vi "StartProgram.vi"(8 "error in (no error)":errorcluster, 11 "FPGA VI Reference In":refnum<k20>) -> (0 "error out":errorcluster, 3 "FPGA VI Reference out":refnum<k20>)   [LabVIEW 2018]
uses:
  Type_Def/Type_Def ControlState.ctl
  Type_Def/Type_Def Master_DataControls.ctl
  Type_Def/TypeDef_cRIODatas.ctl
  Type_Def/Type_Def IMUDatas.ctl
  Type_Def/TypeDef_BMSDatas.ctl
  Type_Def/TypeDef_BMSStatuss.ctl
  Type_Def/TypeDef FixedMotorData.ctl
  Type_Def/Type_Def Actuator Controls.ctl
  Type_Def/TypeDef_MotorData.ctl
  Type_Def/TypeDef_LoopPeriod.ctl
  Type_Def/Master_DataControl.ctl
  <vilib>/Utility/error.llb/Error Cluster From Error Code.vi
  <vilib>/rvi/errors/niLvFpgaAdjustHostInterfaceError.vi
  <vilib>/rvi/interface/nirviReadWriteControl/nirviReadWriteControl.xnode
  <vilib>/NI_Real-Time Target Support.lvlib
  NiFpgaLv.dll
  <vilib>/rvi/interface/Simulation/niFpgaSimulationCallBeginRW.vi
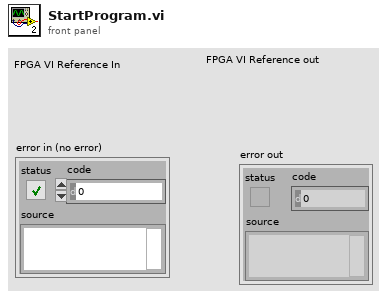
[diagram p1: front panel]
types:
  T1 = cluster{"x acceleration (g)":dbl, "Pressure (psia)":dbl, "Temperature (F)":dbl}
  T2 = typedef "Type_Def Master_DataControls.ctl" = cluster{"cRIO Data":T3, "IMU Data":T4, "BMS Data":T5, "Motor Data":T7}
  T3 = typedef "TypeDef_cRIODatas.ctl" = cluster{"HallEffect Right (cm)":dbl, "HallEffect Left (cm)":dbl, "Optical Sensor 1 (V)":dbl, "Optical Sensor 2 (V)":dbl, "24V Voltage  (V)":dbl, "24V Current (A)":dbl, "Contactor H1 Continuity":dbl, "Contactor L1 Continuity ":dbl, "Contactor H2 Continuity":dbl, "Contactor L2 Continuity ":dbl, "Brake PT(psig)":dbl, "Pump PT (psig)":dbl, "24V Temp   (C)":dbl, "Tank PT(psig) ":dbl, "ABS Pressure 1 (psig)":dbl, "ABS Pressure 2 (psig) ":dbl, "Displacement (ft)":dbl, "Velocity (ft/s)":dbl, "Time (ms)":dbl, "PV 1 Temp":dbl, "PV2 Temp":dbl}
  T4 = typedef "Type_Def IMUDatas.ctl" = cluster{"x acceleration (g)":dbl, "Pressure (psia)":dbl, "Temperature (F)":dbl}
  T5 = typedef "TypeDef_BMSDatas.ctl" = cluster{"Pack 1 Max Cell\n Voltage (V)":dbl, "Pack 1 Max Cell\n ID ":dbl, "Pack 1 Min Cell \nVoltage (V)":dbl, "Pack 1 Min Cell \nID ":dbl, "Pack 1 State of Charge  (%)":dbl, "Pack 1 Average Voltage1 (V)":dbl, "Pack 1Voltage Delta (V)":dbl, "Pack 1 Current (A)":dbl, "Pack 1 Voltage (V)":dbl, "Pack 1 Max Resistance (Ohm)":dbl, "Pack 1Min Resistance (Ohm)":dbl, "Pack 1Average Resistance (Ohm)":dbl, "Pack 1Delta Resistance (Ohm)":dbl, "Pack 1 Highest Temperature(F)":dbl, "BmsStatus1":T6, "Pack 2 Max Cell\n Voltage (V) ":dbl, "Pack 2 Max Cell\n ID  ":dbl, "Pack 2 Min Cell \nVoltage (V) ":dbl, "Pack 2 Min Cell \nID  ":dbl, "Pack 2 Average Voltage1 (V)":dbl, "Pack 2 Voltage Delta (V) ":dbl, "Pack 2 Current (A)":dbl, "Pack 2 Voltage (V) ":dbl, "Pack 2 State of Charge  (%) ":dbl, "Pack 2 Max Resistance (Ohm) ":dbl, "Pack 2 Min Resistance (Ohm)":dbl, "Pack 2 Average Resistance (Ohm)":dbl, "Pack 2 Delta Resistance (Ohm) ":dbl, "Pack 2 Highest Temperature(F) ":dbl, "BmsStatus 2":T6}
  T6 = typedef "TypeDef_BMSStatuss.ctl" = cluster{"isFault":bool, "isolationMonitoring":bool}
  T7 = typedef "TypeDef FixedMotorData.ctl" = cluster{" Velocity (RPM)":dbl, " MotorTemp(C)":dbl, " ControlTemp(C)":dbl, " DcLinkVolt(V)":dbl, " ErrorCode":dbl, "IsAlive":bool, "motorStatus":cluster{"isReady":bool, "isOn":bool, "isOperEn":bool, "isFault":bool, "isVoltEn":bool, "targetReached":bool, "isWarning":bool}, "motorControllerState":u16}
  T8 = typedef "TypeDef_MotorData.ctl" = cluster{" Velocity (RPM)":i32, " MotorTemp(C)":u8, " ControlTemp(C)":u8, " DcLinkVolt(V)":dbl, " ErrorCode":dbl, "IsAlive":bool, "motorStatus":cluster{"isReady":bool, "isOn":bool, "isOperEn":bool, "isFault":bool, "isVoltEn":bool, "targetReached":bool, "isWarning":bool}, "motorControllerState":u16}
  T9 = typedef "Type_Def Actuator Controls.ctl" = cluster{"Reverse ":bool, "Precharge Ctrl":bool, "Pump Ctrl":bool, "24 VDC Ctr":bool, "Vent Solenoid":bool, "Brake Solenoid":bool, "EMCY  Brake Solenoid":bool, "Digital Out 7B ":bool, "Forward Ctrl":bool, "Contact H1":bool, "Contact L1":bool, "Contact H2":bool, "Contact L2 ":bool, "LED RED":bool, "LED GREEN":bool, " Digital Out 7A":bool}
  T10 = typedef "Type_Def ControlState.ctl" = enum16{"Blank", "Systems Check", "Idle", "Ready", "Pushing", "CrawlingPrecharge", "Braking", "Fault", "Boot Up", "Unpowered", "Crawling", "Shutdown", "Service Push", "Service Wait", "Vent", "Precharge"}
  T11 = cluster{"Forward":bool, "Low Side":bool, "Precharge":bool, "High Side":bool, "Digital Out 5":bool, "Digital Out 6":bool, "Digital Out 7 ":bool, "24 Power":bool, "Tank Valve ":bool, "Brake Valve":bool, "Pump":bool, "Digital Out 1 ":bool, "Digital Out 2":bool, "Digital Out 3":bool, "Digital Out 4 ":bool, "Reverse":bool}
  T12 = typedef "TypeDef_LoopPeriod.ctl" = cluster{"Control Period":i64, "DAQ Period":u32, "IMU Period":u32, "CAN Period":i64, "Nav Period":u32}
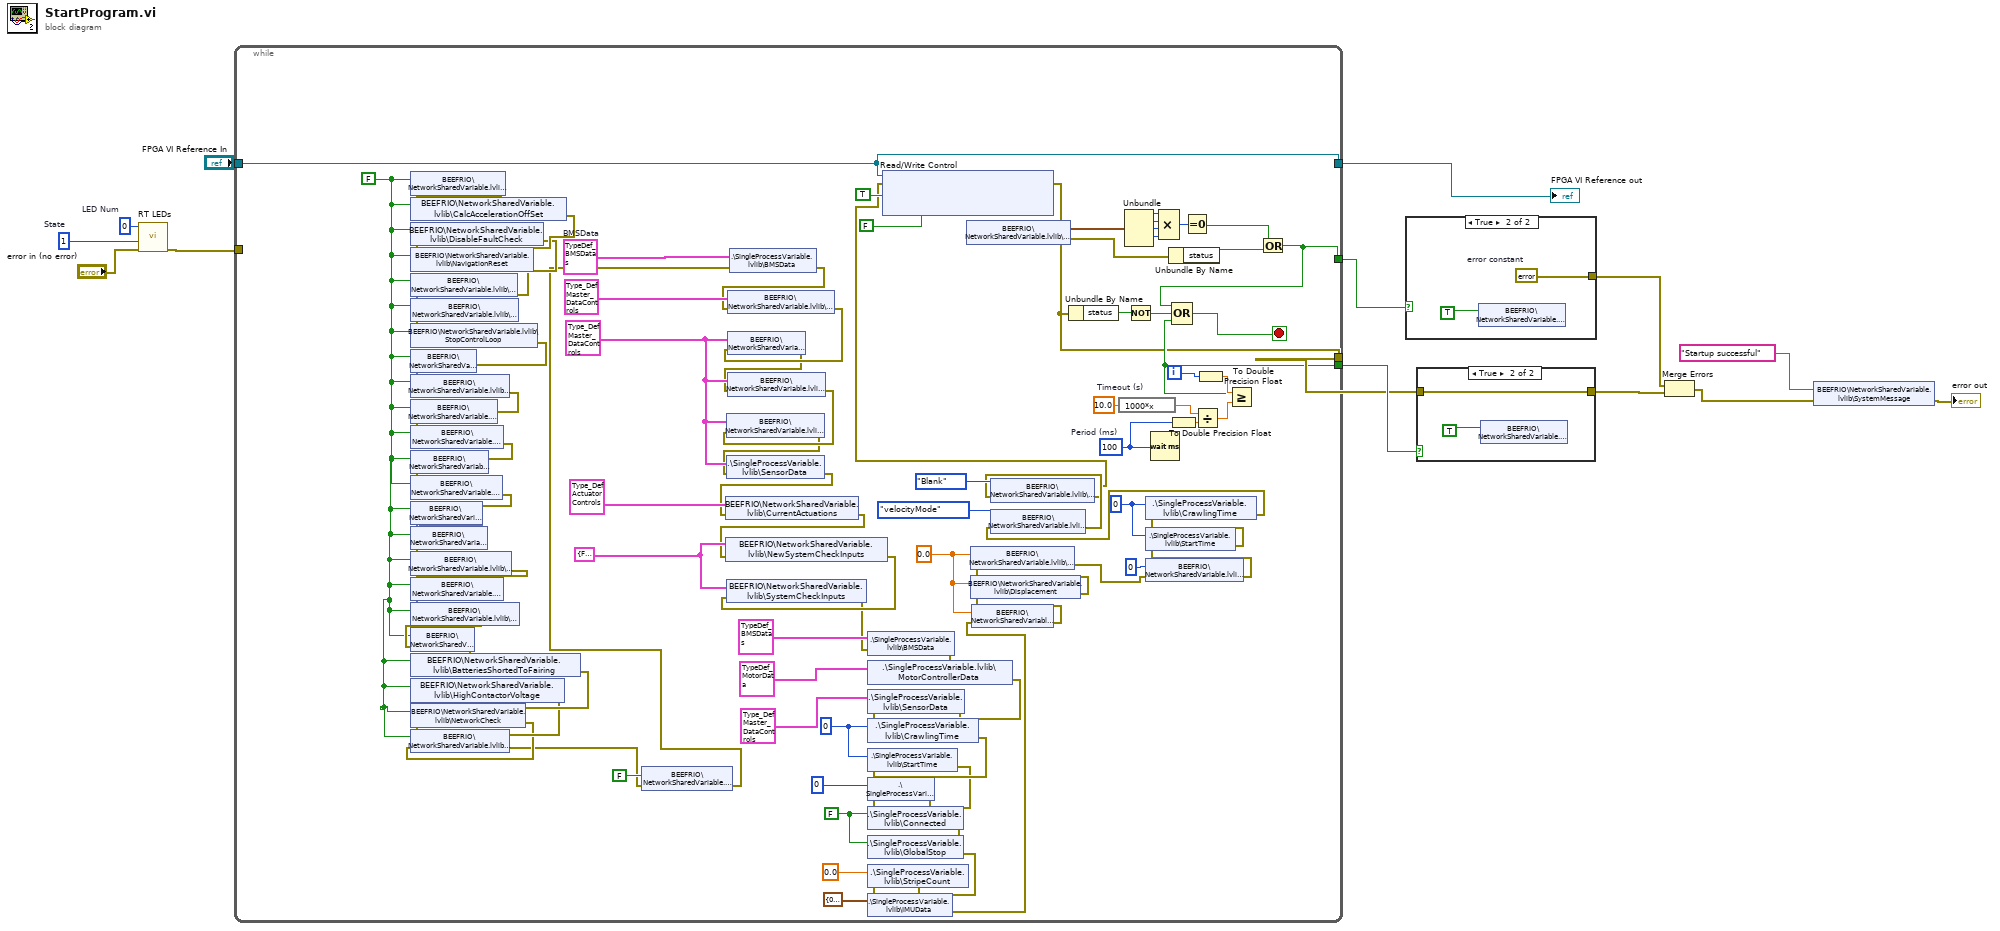
[diagram p0: block diagram]
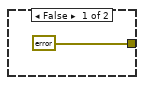
[diagram p2: hidden frame]
diagram:
  w11 = 1  # State
  w12 = 0  # LED Num
  n1 = call <vilib>:"RT LEDs.vi"("error in (no error)"="error in (no error)", "State"=w11, "LED Num"=w12) -> ("error out"=w9:errorcluster)  [unwired: 3 in, 1 out]
  n2 = while {
    tunnel: [w108] -> w14
    tunnel: "FPGA VI Reference In" -> [w108]
    tunnel: w9 -> [_]
    tunnel: [w43] -> w8
    tunnel: [w89] -> w7
    tunnel: [w87] -> w6
    i -> [w88]
    stop <- w90 stop-if-true
    w72 = FALSE ("Connected")
    w73 = i64 0 ("CrawlingTime")
    w77 = T11 {"Forward"=FALSE, "Low Side"=FALSE, "Precharge"=FALSE, "High Side"=FALSE, "Digital Out 5"=FALSE, "Digital Out 6"=FALSE, "Digital Out 7 "=FALSE, "24 Power"=FALSE, "Tank Valve "=FALSE, "Brake Valve"=FALSE, "Pump"=FALSE, "Digital Out 1 "=FALSE, "Digital Out 2"=FALSE, "Digital Out 3"=FALSE, "Digital Out 4 "=FALSE, "Reverse"=FALSE} ("NewSystemCheckInputs")
    w79 = T2 {"cRIO Data"={"HallEffect Right (cm)"=0.0, "HallEffect Left (cm)"=0.0, "Optical Sensor 1 (V)"=0.0, "Optical Sensor 2 (V)"=0.0, "24V Voltage  (V)"=0.0, "24V Current (A)"=0.0, "Contactor H1 Continuity"=0.0, "Contactor L1 Continuity "=0.0, "Contactor H2 Continuity"=0.0, "Contactor L2 Continuity "=0.0, "Brake PT(psig)"=0.0, "Pump PT (psig)"=0.0, "24V Temp   (C)"=0.0, "Tank PT(psig) "=0.0, "ABS Pressure 1 (psig)"=0.0, "ABS Pressure 2 (psig) "=0.0, "Displacement (ft)"=0.0, "Velocity (ft/s)"=0.0, "Time (ms)"=0.0, "PV 1 Temp"=0.0, "PV2 Temp"=0.0}, "IMU Data"={"x acceleration (g)"=0.0, "Pressure (psia)"=0.0, "Temperature (F)"=0.0}, "BMS Data"={"Pack 1 Max Cell\n Voltage (V)"=0.0, "Pack 1 Max Cell\n ID "=0.0, "Pack 1 Min Cell \nVoltage (V)"=0.0, "Pack 1 Min Cell \nID "=0.0, "Pack 1 State of Charge  (%)"=0.0, "Pack 1 Average Voltage1 (V)"=0.0, "Pack 1Voltage Delta (V)"=0.0, "Pack 1 Current (A)"=0.0, "Pack 1 Voltage (V)"=0.0, "Pack 1 Max Resistance (Ohm)"=0.0, "Pack 1Min Resistance (Ohm)"=0.0, "Pack 1Average Resistance (Ohm)"=0.0, "Pack 1Delta Resistance (Ohm)"=0.0, "Pack 1 Highest Temperature(F)"=0.0, "BmsStatus1"={"isFault"=FALSE, "isolationMonitoring"=FALSE}, "Pack 2 Max Cell\n Voltage (V) "=0.0, "Pack 2 Max Cell\n ID  "=0.0, "Pack 2 Min Cell \nVoltage (V) "=0.0, "Pack 2 Min Cell \nID  "=0.0, "Pack 2 Average Voltage1 (V)"=0.0, "Pack 2 Voltage Delta (V) "=0.0, "Pack 2 Current (A)"=0.0, "Pack 2 Voltage (V) "=0.0, "Pack 2 State of Charge  (%) "=0.0, "Pack 2 Max Resistance (Ohm) "=0.0, "Pack 2 Min Resistance (Ohm)"=0.0, "Pack 2 Average Resistance (Ohm)"=0.0, "Pack 2 Delta Resistance (Ohm) "=0.0, "Pack 2 Highest Temperature(F) "=0.0, "BmsStatus 2"={"isFault"=FALSE, "isolationMonitoring"=FALSE}}, "Motor Data"={" Velocity (RPM)"=0.0, " MotorTemp(C)"=0.0, " ControlTemp(C)"=0.0, " DcLinkVolt(V)"=0.0, " ErrorCode"=0.0, "IsAlive"=FALSE, "motorStatus"={"isReady"=FALSE, "isOn"=FALSE, "isOperEn"=FALSE, "isFault"=FALSE, "isVoltEn"=FALSE, "targetReached"=FALSE, "isWarning"=FALSE}, "motorControllerState"=1}} ("AllData")
    w81 = T5 {"Pack 1 Max Cell\n Voltage (V)"=0.0, "Pack 1 Max Cell\n ID "=0.0, "Pack 1 Min Cell \nVoltage (V)"=0.0, "Pack 1 Min Cell \nID "=0.0, "Pack 1 State of Charge  (%)"=0.0, "Pack 1 Average Voltage1 (V)"=0.0, "Pack 1Voltage Delta (V)"=0.0, "Pack 1 Current (A)"=0.0, "Pack 1 Voltage (V)"=0.0, "Pack 1 Max Resistance (Ohm)"=0.0, "Pack 1Min Resistance (Ohm)"=0.0, "Pack 1Average Resistance (Ohm)"=0.0, "Pack 1Delta Resistance (Ohm)"=0.0, "Pack 1 Highest Temperature(F)"=0.0, "BmsStatus1"={"isFault"=FALSE, "isolationMonitoring"=FALSE}, "Pack 2 Max Cell\n Voltage (V) "=0.0, "Pack 2 Max Cell\n ID  "=0.0, "Pack 2 Min Cell \nVoltage (V) "=0.0, "Pack 2 Min Cell \nID  "=0.0, "Pack 2 Average Voltage1 (V)"=0.0, "Pack 2 Voltage Delta (V) "=0.0, "Pack 2 Current (A)"=0.0, "Pack 2 Voltage (V) "=0.0, "Pack 2 State of Charge  (%) "=0.0, "Pack 2 Max Resistance (Ohm) "=0.0, "Pack 2 Min Resistance (Ohm)"=0.0, "Pack 2 Average Resistance (Ohm)"=0.0, "Pack 2 Delta Resistance (Ohm) "=0.0, "Pack 2 Highest Temperature(F) "=0.0, "BmsStatus 2"={"isFault"=FALSE, "isolationMonitoring"=FALSE}}  # BMSData
    w82 = 0.0 ("Acceleration")
    w17 = FALSE ("BMSFreeze")
    w105 = 10.0  # Timeout (s)
    w103 = u32 100  # Period (ms)
    w86 = i64 0 ("StartTime")
    n3 = shared-variable "BEEFRIO\\NetworkSharedVariable.lvlib\\BMSFreeze"(w17) -> (error out=w69:errorcluster)  [unwired: 1 in]
    n4 = shared-variable "BEEFRIO\\NetworkSharedVariable.lvlib\\CalcAccelerationOffSet"(w17, error in=w69) -> (error out=w68:errorcluster)
    n5 = shared-variable "BEEFRIO\\NetworkSharedVariable.lvlib\\DisableFaultCheck"(w17, error in=w68) -> (error out=w67:errorcluster)
    n6 = shared-variable "BEEFRIO\\NetworkSharedVariable.lvlib\\NavigationReset"(w17, error in=w67) -> (error out=w66:errorcluster)
    n7 = shared-variable "BEEFRIO\\NetworkSharedVariable.lvlib\\ReIntStreams"(w17, error in=w66) -> (error out=w65:errorcluster)
    n8 = shared-variable "BEEFRIO\\NetworkSharedVariable.lvlib\\SimulateData"(w17, error in=w65) -> (error out=w64:errorcluster)
    n9 = shared-variable "BEEFRIO\\NetworkSharedVariable.lvlib\\StopControlLoop"(w17, error in=w64) -> (error out=w63:errorcluster)
    n10 = shared-variable "BEEFRIO\\NetworkSharedVariable.lvlib\\Fault"(w17, error in=w63) -> (error out=w62:errorcluster)
    n11 = shared-variable "BEEFRIO\\NetworkSharedVariable.lvlib\\driveEnable"(w17, error in=w62) -> (error out=w61:errorcluster)
    n12 = shared-variable "BEEFRIO\\NetworkSharedVariable.lvlib\\ForceIdle"(w17, error in=w61) -> (error out=w60:errorcluster)
    n13 = shared-variable "BEEFRIO\\NetworkSharedVariable.lvlib\\IsPowered"(w17, error in=w60) -> (error out=w59:errorcluster)
    n14 = shared-variable "BEEFRIO\\NetworkSharedVariable.lvlib\\Launch"(w17, error in=w59) -> (error out=w58:errorcluster)
    n15 = shared-variable "BEEFRIO\\NetworkSharedVariable.lvlib\\Precharge"(w17, error in=w58) -> (error out=w57:errorcluster)
    n16 = shared-variable "BEEFRIO\\NetworkSharedVariable.lvlib\\Ready"(w17, error in=w57) -> (error out=w56:errorcluster)
    n17 = shared-variable "BEEFRIO\\NetworkSharedVariable.lvlib\\Service"(w17, error in=w56) -> (error out=w55:errorcluster)
    n18 = shared-variable "BEEFRIO\\NetworkSharedVariable.lvlib\\ServicePush"(w17, error in=w55) -> (error out=w54:errorcluster)
    n19 = shared-variable "BEEFRIO\\NetworkSharedVariable.lvlib\\Shutdown"(w17, error in=w54) -> (error out=w53:errorcluster)
    n20 = shared-variable "BEEFRIO\\NetworkSharedVariable.lvlib\\SystemCheck"(w17, error in=w53) -> (error out=w52:errorcluster)
    n21 = shared-variable "BEEFRIO\\NetworkSharedVariable.lvlib\\Vent"(w17, error in=w52) -> (error out=w21:errorcluster)
    n22 = shared-variable "BEEFRIO\\NetworkSharedVariable.lvlib\\BatteriesShortedToFairing"(w17, error in=w21) -> (error out=w20:errorcluster)
    n23 = shared-variable "BEEFRIO\\NetworkSharedVariable.lvlib\\HighContactorVoltage"(w17, error in=w20) -> (error out=w19:errorcluster)
    n24 = shared-variable "BEEFRIO\\NetworkSharedVariable.lvlib\\NetworkCheck"(w17, error in=w19) -> (error out=w18:errorcluster)
    n25 = shared-variable "BEEFRIO\\NetworkSharedVariable.lvlib\\driveEnable"(w17, error in=w18) -> (error out=w16:errorcluster)
    n26 = shared-variable "BEEFRIO\\NetworkSharedVariable.lvlib\\ReintCAN"(FALSE ("ReintCAN"), error in=w16) -> (error out=w15:errorcluster)
    n27 = shared-variable ".\\SingleProcessVariable.lvlib\\BMSData"(w81, error in=w15) -> (error out=w51:errorcluster)
    n28 = shared-variable "BEEFRIO\\NetworkSharedVariable.lvlib\\DataOverride"(T2 {"cRIO Data"={"HallEffect Right (cm)"=0.0, "HallEffect Left (cm)"=0.0, "Optical Sensor 1 (V)"=0.0, "Optical Sensor 2 (V)"=0.0, "24V Voltage  (V)"=0.0, "24V Current (A)"=0.0, "Contactor H1 Continuity"=0.0, "Contactor L1 Continuity "=0.0, "Contactor H2 Continuity"=0.0, "Contactor L2 Continuity "=0.0, "Brake PT(psig)"=0.0, "Pump PT (psig)"=0.0, "24V Temp   (C)"=0.0, "Tank PT(psig) "=0.0, "ABS Pressure 1 (psig)"=0.0, "ABS Pressure 2 (psig) "=0.0, "Displacement (ft)"=0.0, "Velocity (ft/s)"=0.0, "Time (ms)"=0.0, "PV 1 Temp"=0.0, "PV2 Temp"=0.0}, "IMU Data"={"x acceleration (g)"=0.0, "Pressure (psia)"=0.0, "Temperature (F)"=0.0}, "BMS Data"={"Pack 1 Max Cell\n Voltage (V)"=0.0, "Pack 1 Max Cell\n ID "=0.0, "Pack 1 Min Cell \nVoltage (V)"=0.0, "Pack 1 Min Cell \nID "=0.0, "Pack 1 State of Charge  (%)"=0.0, "Pack 1 Average Voltage1 (V)"=0.0, "Pack 1Voltage Delta (V)"=0.0, "Pack 1 Current (A)"=0.0, "Pack 1 Voltage (V)"=0.0, "Pack 1 Max Resistance (Ohm)"=0.0, "Pack 1Min Resistance (Ohm)"=0.0, "Pack 1Average Resistance (Ohm)"=0.0, "Pack 1Delta Resistance (Ohm)"=0.0, "Pack 1 Highest Temperature(F)"=0.0, "BmsStatus1"={"isFault"=FALSE, "isolationMonitoring"=FALSE}, "Pack 2 Max Cell\n Voltage (V) "=0.0, "Pack 2 Max Cell\n ID  "=0.0, "Pack 2 Min Cell \nVoltage (V) "=0.0, "Pack 2 Min Cell \nID  "=0.0, "Pack 2 Average Voltage1 (V)"=0.0, "Pack 2 Voltage Delta (V) "=0.0, "Pack 2 Current (A)"=0.0, "Pack 2 Voltage (V) "=0.0, "Pack 2 State of Charge  (%) "=0.0, "Pack 2 Max Resistance (Ohm) "=0.0, "Pack 2 Min Resistance (Ohm)"=0.0, "Pack 2 Average Resistance (Ohm)"=0.0, "Pack 2 Delta Resistance (Ohm) "=0.0, "Pack 2 Highest Temperature(F) "=0.0, "BmsStatus 2"={"isFault"=FALSE, "isolationMonitoring"=FALSE}}, "Motor Data"={" Velocity (RPM)"=0.0, " MotorTemp(C)"=0.0, " ControlTemp(C)"=0.0, " DcLinkVolt(V)"=0.0, " ErrorCode"=0.0, "IsAlive"=FALSE, "motorStatus"={"isReady"=FALSE, "isOn"=FALSE, "isOperEn"=FALSE, "isFault"=FALSE, "isVoltEn"=FALSE, "targetReached"=FALSE, "isWarning"=FALSE}, "motorControllerState"=1}} ("DataOverride"), error in=w51) -> (error out=w50:errorcluster)
    n29 = shared-variable "BEEFRIO\\NetworkSharedVariable.lvlib\\AllData"(w79, error in=w50) -> (error out=w49:errorcluster)
    n30 = shared-variable "BEEFRIO\\NetworkSharedVariable.lvlib\\AllDataMax"(w79, error in=w49) -> (error out=w48:errorcluster)
    n31 = shared-variable "BEEFRIO\\NetworkSharedVariable.lvlib\\AllDataMin"(w79, error in=w48) -> (error out=w47:errorcluster)
    n32 = shared-variable ".\\SingleProcessVariable.lvlib\\SensorData"(w79, error in=w47) -> (error out=w46:errorcluster)
    n33 = shared-variable "BEEFRIO\\NetworkSharedVariable.lvlib\\CurrentActuations"(T9 {"Reverse "=FALSE, "Precharge Ctrl"=FALSE, "Pump Ctrl"=FALSE, "24 VDC Ctr"=FALSE, "Vent Solenoid"=FALSE, "Brake Solenoid"=FALSE, "EMCY  Brake Solenoid"=FALSE, "Digital Out 7B "=FALSE, "Forward Ctrl"=FALSE, "Contact H1"=FALSE, "Contact L1"=FALSE, "Contact H2"=FALSE, "Contact L2 "=FALSE, "LED RED"=FALSE, "LED GREEN"=FALSE, " Digital Out 7A"=FALSE} ("CurrentActuations"), error in=w46) -> (error out=w45:errorcluster)
    n34 = shared-variable "BEEFRIO\\NetworkSharedVariable.lvlib\\NewSystemCheckInputs"(w77, error in=w45) -> (error out=w44:errorcluster)
    n35 = shared-variable "BEEFRIO\\NetworkSharedVariable.lvlib\\SystemCheckInputs"(w77, error in=w44) -> (error out=w42:errorcluster)
    n36 = shared-variable ".\\SingleProcessVariable.lvlib\\BMSData"(T5 {"Pack 1 Max Cell\n Voltage (V)"=0.0, "Pack 1 Max Cell\n ID "=0.0, "Pack 1 Min Cell \nVoltage (V)"=0.0, "Pack 1 Min Cell \nID "=0.0, "Pack 1 State of Charge  (%)"=0.0, "Pack 1 Average Voltage1 (V)"=0.0, "Pack 1Voltage Delta (V)"=0.0, "Pack 1 Current (A)"=0.0, "Pack 1 Voltage (V)"=0.0, "Pack 1 Max Resistance (Ohm)"=0.0, "Pack 1Min Resistance (Ohm)"=0.0, "Pack 1Average Resistance (Ohm)"=0.0, "Pack 1Delta Resistance (Ohm)"=0.0, "Pack 1 Highest Temperature(F)"=0.0, "BmsStatus1"={"isFault"=FALSE, "isolationMonitoring"=FALSE}, "Pack 2 Max Cell\n Voltage (V) "=0.0, "Pack 2 Max Cell\n ID  "=0.0, "Pack 2 Min Cell \nVoltage (V) "=0.0, "Pack 2 Min Cell \nID  "=0.0, "Pack 2 Average Voltage1 (V)"=0.0, "Pack 2 Voltage Delta (V) "=0.0, "Pack 2 Current (A)"=0.0, "Pack 2 Voltage (V) "=0.0, "Pack 2 State of Charge  (%) "=0.0, "Pack 2 Max Resistance (Ohm) "=0.0, "Pack 2 Min Resistance (Ohm)"=0.0, "Pack 2 Average Resistance (Ohm)"=0.0, "Pack 2 Delta Resistance (Ohm) "=0.0, "Pack 2 Highest Temperature(F) "=0.0, "BmsStatus 2"={"isFault"=FALSE, "isolationMonitoring"=FALSE}} ("BMSData"), error in=w42) -> (error out=w41:errorcluster)
    n37 = shared-variable ".\\SingleProcessVariable.lvlib\\MotorControllerData"(T8 {" Velocity (RPM)"=0, " MotorTemp(C)"=0, " ControlTemp(C)"=0, " DcLinkVolt(V)"=0.0, " ErrorCode"=0.0, "IsAlive"=FALSE, "motorStatus"={"isReady"=FALSE, "isOn"=FALSE, "isOperEn"=FALSE, "isFault"=FALSE, "isVoltEn"=FALSE, "targetReached"=FALSE, "isWarning"=FALSE}, "motorControllerState"=1} ("MotorControllerData"), error in=w41) -> (error out=w40:errorcluster)
    n38 = shared-variable ".\\SingleProcessVariable.lvlib\\SensorData"(T2 {"cRIO Data"={"HallEffect Right (cm)"=0.0, "HallEffect Left (cm)"=0.0, "Optical Sensor 1 (V)"=0.0, "Optical Sensor 2 (V)"=0.0, "24V Voltage  (V)"=0.0, "24V Current (A)"=0.0, "Contactor H1 Continuity"=0.0, "Contactor L1 Continuity "=0.0, "Contactor H2 Continuity"=0.0, "Contactor L2 Continuity "=0.0, "Brake PT(psig)"=0.0, "Pump PT (psig)"=0.0, "24V Temp   (C)"=0.0, "Tank PT(psig) "=0.0, "ABS Pressure 1 (psig)"=0.0, "ABS Pressure 2 (psig) "=0.0, "Displacement (ft)"=0.0, "Velocity (ft/s)"=0.0, "Time (ms)"=0.0, "PV 1 Temp"=0.0, "PV2 Temp"=0.0}, "IMU Data"={"x acceleration (g)"=0.0, "Pressure (psia)"=0.0, "Temperature (F)"=0.0}, "BMS Data"={"Pack 1 Max Cell\n Voltage (V)"=0.0, "Pack 1 Max Cell\n ID "=0.0, "Pack 1 Min Cell \nVoltage (V)"=0.0, "Pack 1 Min Cell \nID "=0.0, "Pack 1 State of Charge  (%)"=0.0, "Pack 1 Average Voltage1 (V)"=0.0, "Pack 1Voltage Delta (V)"=0.0, "Pack 1 Current (A)"=0.0, "Pack 1 Voltage (V)"=0.0, "Pack 1 Max Resistance (Ohm)"=0.0, "Pack 1Min Resistance (Ohm)"=0.0, "Pack 1Average Resistance (Ohm)"=0.0, "Pack 1Delta Resistance (Ohm)"=0.0, "Pack 1 Highest Temperature(F)"=0.0, "BmsStatus1"={"isFault"=FALSE, "isolationMonitoring"=FALSE}, "Pack 2 Max Cell\n Voltage (V) "=0.0, "Pack 2 Max Cell\n ID  "=0.0, "Pack 2 Min Cell \nVoltage (V) "=0.0, "Pack 2 Min Cell \nID  "=0.0, "Pack 2 Average Voltage1 (V)"=0.0, "Pack 2 Voltage Delta (V) "=0.0, "Pack 2 Current (A)"=0.0, "Pack 2 Voltage (V) "=0.0, "Pack 2 State of Charge  (%) "=0.0, "Pack 2 Max Resistance (Ohm) "=0.0, "Pack 2 Min Resistance (Ohm)"=0.0, "Pack 2 Average Resistance (Ohm)"=0.0, "Pack 2 Delta Resistance (Ohm) "=0.0, "Pack 2 Highest Temperature(F) "=0.0, "BmsStatus 2"={"isFault"=FALSE, "isolationMonitoring"=FALSE}}, "Motor Data"={" Velocity (RPM)"=0.0, " MotorTemp(C)"=0.0, " ControlTemp(C)"=0.0, " DcLinkVolt(V)"=0.0, " ErrorCode"=0.0, "IsAlive"=FALSE, "motorStatus"={"isReady"=FALSE, "isOn"=FALSE, "isOperEn"=FALSE, "isFault"=FALSE, "isVoltEn"=FALSE, "targetReached"=FALSE, "isWarning"=FALSE}, "motorControllerState"=1}} ("SensorData"), error in=w40) -> (error out=w39:errorcluster)
    n39 = shared-variable ".\\SingleProcessVariable.lvlib\\CrawlingTime"(w73, error in=w39) -> (error out=w38:errorcluster)
    n40 = shared-variable ".\\SingleProcessVariable.lvlib\\StartTime"(w73, error in=w38) -> (error out=w37:errorcluster)
    n41 = shared-variable ".\\SingleProcessVariable.lvlib\\Time"(i64 0 ("Time"), error in=w37) -> (error out=w36:errorcluster)
    n42 = shared-variable ".\\SingleProcessVariable.lvlib\\Connected"(w72, error in=w36) -> (error out=w35:errorcluster)
    n43 = shared-variable ".\\SingleProcessVariable.lvlib\\GlobalStop"(w72, error in=w35) -> (error out=w34:errorcluster)
    n44 = shared-variable ".\\SingleProcessVariable.lvlib\\StripeCount"(0.0 ("StripeCount"), error in=w34) -> (error out=w33:errorcluster)
    n45 = shared-variable ".\\SingleProcessVariable.lvlib\\IMUData"(T1 {"x acceleration (g)"=0.0, "Pressure (psia)"=0.0, "Temperature (F)"=0.0} ("IMUData"), error in=w33) -> (error out=w31:errorcluster)
    n46 = shared-variable "BEEFRIO\\NetworkSharedVariable.lvlib\\LoopPeriods"() -> (w99:T12, error out=w93:errorcluster)  [unwired: 1 in]
    n47 = shared-variable "BEEFRIO\\NetworkSharedVariable.lvlib\\Velocity"(w82, error in=w31) -> (error out=w30:errorcluster)
    n48 = shared-variable "BEEFRIO\\NetworkSharedVariable.lvlib\\Displacement"(w82, error in=w30) -> (error out=w29:errorcluster)
    n49 = shared-variable "BEEFRIO\\NetworkSharedVariable.lvlib\\Acceleration"(w82, error in=w29) -> (error out=w28:errorcluster)
    n50 = expression code="1000*x"(w105) -> (w104:dbl)
    n51 = Unbundle(w99) -> ("Control Period"=w95:i64, "DAQ Period"=w97:u32, "IMU Period"=w96:u32, "CAN Period"=w98:i64)  [unwired: 1 out]
    n52 = shared-variable "BEEFRIO\\NetworkSharedVariable.lvlib\\driveTarget"(i16 0 ("driveTarget"), error in=w28) -> (error out=w27:errorcluster)
    n53 = shared-variable ".\\SingleProcessVariable.lvlib\\StartTime"(w86, error in=w27) -> (error out=w26:errorcluster)
    n54 = shared-variable ".\\SingleProcessVariable.lvlib\\CrawlingTime"(w86, error in=w26) -> (error out=w25:errorcluster)
    n55 = shared-variable "BEEFRIO\\NetworkSharedVariable.lvlib\\driveMode"(enum16{"velocityMode", "torqueMode", ""}."velocityMode" ("driveMode"), error in=w25) -> (error out=w24:errorcluster)
    n56 = shared-variable "BEEFRIO\\NetworkSharedVariable.lvlib\\CurrentState"(Type_Def_ControlState."Blank" ("CurrentState"), error in=w24) -> (error out=w23:errorcluster)
    n57 = xnode "Read/Write Control"("FPGA VI Reference In"=w108, "error in"=w23, "Enable RT Watchdog"=TRUE ("Boolean"), "RT Reset on Watchdog Failure?"=FALSE) -> ("error out"=w87:errorcluster)  [unwired: 1 out]
    n58 = Unbundle By Name(w87) -> ("status"=w107:bool)
    n59 = Not(x=w107) -> (.not. x?=w106:bool)
    n60 = Wait (ms)(milliseconds to wait=w103) -> ()  [unwired: 1 out]
    n61 = Compound Arithmetic op=MULTIPLY(w95, w97, w96, w98) -> (w94:i64)
    n62 = Unbundle By Name(w93) -> ("status"=w91:bool)
    n63 = To Double Precision Float(number=w103) -> (double precision float=w101:dbl)
    n64 = Equal To 0?(x=w94) -> (x = 0?=w92:bool)
    n65 = Divide(x=w104, y=w101) -> (x/y=w102:dbl)
    n66 = To Double Precision Float(number=w88) -> (double precision float=w100:dbl)
    n67 = Greater Or Equal?(x=w100, y=w102) -> (x >= y?=w89:bool)
    n68 = Or(x=w92, y=w91) -> (x .or. y?=w43:bool)
    n69 = Compound Arithmetic op=OR(w43, w106, w89) -> (w90:bool)
  }
  "FPGA VI Reference out" <- w14
  n70 = case shown="True" w8 {
    tunnel: [errorcluster {"status"=FALSE, "code"=0, "source"=""} ("error constant") w112] -> w4
    frame False {
    }
    frame True {
      w112 = errorcluster {"status"=TRUE, "code"=0, "source"="Loop Periods not set"}  # error constant
      n71 = shared-variable "BEEFRIO\\NetworkSharedVariable.lvlib\\ForceIdle"(TRUE ("Boolean")) -> ()  [unwired: 1 in, 1 out]
    }
  }
  n72 = case shown="True" w7 {
    tunnel: w6 -> [w114 w115]
    tunnel: [w114 w115] -> w5
    frame False {
    }
    frame True {
      n73 = shared-variable "BEEFRIO\\NetworkSharedVariable.lvlib\\ForceIdle"(TRUE ("Boolean")) -> ()  [unwired: 1 in, 1 out]
    }
  }
  n74 = Merge Errors(w4, w5) -> (w1:errorcluster)
  n75 = shared-variable "BEEFRIO\\NetworkSharedVariable.lvlib\\SystemMessage"("Startup successful" ("SysMessage"), error in=w1) -> (error out=→"error out":errorcluster)
